vi "Configuracion inicial de Lock-IN.vi"(2 "error in (no error)":errorcluster, 3 "VISA resource name":refnum<visa-resource-name>) -> (0 "error out":errorcluster, 1 "VISA resource name out":refnum<visa-resource-name>)   [LabVIEW 2018]
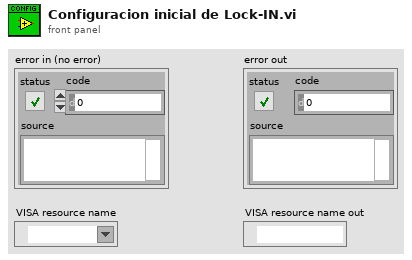
[diagram p1: front panel]
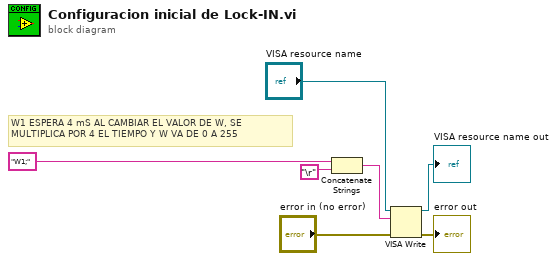
[diagram p0: block diagram]
diagram:
  # "W1 ESPERA 4 mS AL CAMBIAR EL VALOR DE W, SE MULTIPLICA POR 4 EL TIEMPO Y W VA DE 0 A 255"
  n1 = Concatenate Strings("W1;" ("string"), "\r") -> (w7:string)
  n2 = VISA Write(VISA resource name="VISA resource name", write buffer=w7, error in (no error)="error in (no error)") -> (VISA resource name out=→"VISA resource name out":refnum<visa-resource-name>, error out=→"error out":errorcluster)  [unwired: 1 out]
